vi "Position.vi"() -> ()   [LabVIEW 2019]
panel:
  in  "VISA Resource Name Barcode":refnum<visa-resource-name>
  in  "VISA Resource Name AI Motor":refnum<visa-resource-name>
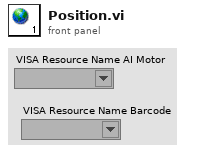
[diagram p1: front panel]
diagram:
